vi "Main.vi"() -> ()   [LabVIEW 2014]
doc: "该连续测量范例项目在队列消息处理器模板的基础上实现。\n\n事件处理循环负责按用户界面操作生成对应的消息。\n\n消息处理循环负责对事件处理循环或其他消息生成的消息进行处理。其中还包括用于采集和记录消息处理循环的子VI，以及用于更新图表的循环。"
uses:
  Settings/Settings.ctl
  Acquisition/Hardware Configuration.ctl
  Acquisition/Signal Type.ctl
  Logging/Logging Configuration.ctl
  controls/UI Data.ctl
  controls/UI State.ctl
  support/Message Queue/Enqueue Message (Single).vi
  support/Message Queue/Enqueue Message (Array).vi
  <vilib>/Utility/error.llb/Error Cluster From Error Code.vi
  <vilib>/ErrorRing/Error Ring.xnode
  Acquisition/Acquisition.lvlib
  Logging/Logging.lvlib
  Settings/Settings.lvlib
  support/User Event - Stop/User Event - Stop.lvlib
  support/Message Queue/Message Queue.lvlib
panel:
  out "数据":waveform(dbl)[](graph)
  in  "设置":bool
  in  "开始":bool
  in  "停止":bool
  out "状态":string
  in  "退出":bool
  # "连续测量数据记录器"
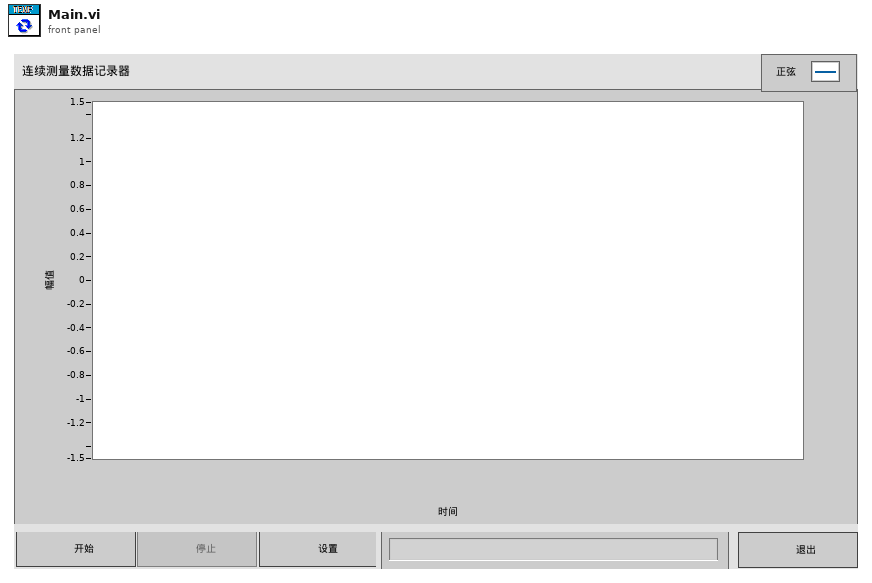
[diagram p1: front panel]
types:
  T1 = typedef "UI State.ctl" = enum16{"Idle", "Acquiring and Logging", "Waiting for Exit", "Waiting for Exit (Acq Stopped)", "Waiting for Exit (Log Stopped)", "Waiting for Stop", "Waiting for Stop (Acq Stopped)", "Waiting for Stop (Log Stopped)"}
  T2 = typedef "UI Data.ctl" = cluster{"开始引用":refnum<vi>, "停止引用":refnum<vi>, "设置引用":refnum<vi>, "退出引用":refnum<vi>, "状态引用":refnum<vi>, "数据引用":refnum<vi>}
  T3 = typedef "Settings.lvlib/Settings.ctl" = cluster{"硬件配置":T4, "记录配置":T6}
  T4 = typedef "Acquisition.lvlib/Hardware Configuration.ctl" = cluster{"硬件引用句柄<替换此项>":string, "信号类型<替换该项>":T5}
  T5 = typedef "Acquisition.lvlib/Signal Type.ctl" = enum16{"Sine Wave", "Square with Noise"}
  T6 = typedef "Logging.lvlib/Logging Configuration.ctl" = cluster{"记录文件基路径":path, "TDMS文件引用":refnum<k34>}
  T7 = typedef "Message Queue.lvlib/All Message Queues.ctl" = cluster{"UI":refnum<queue>, "采集":refnum<queue>, "记录":refnum<queue>}
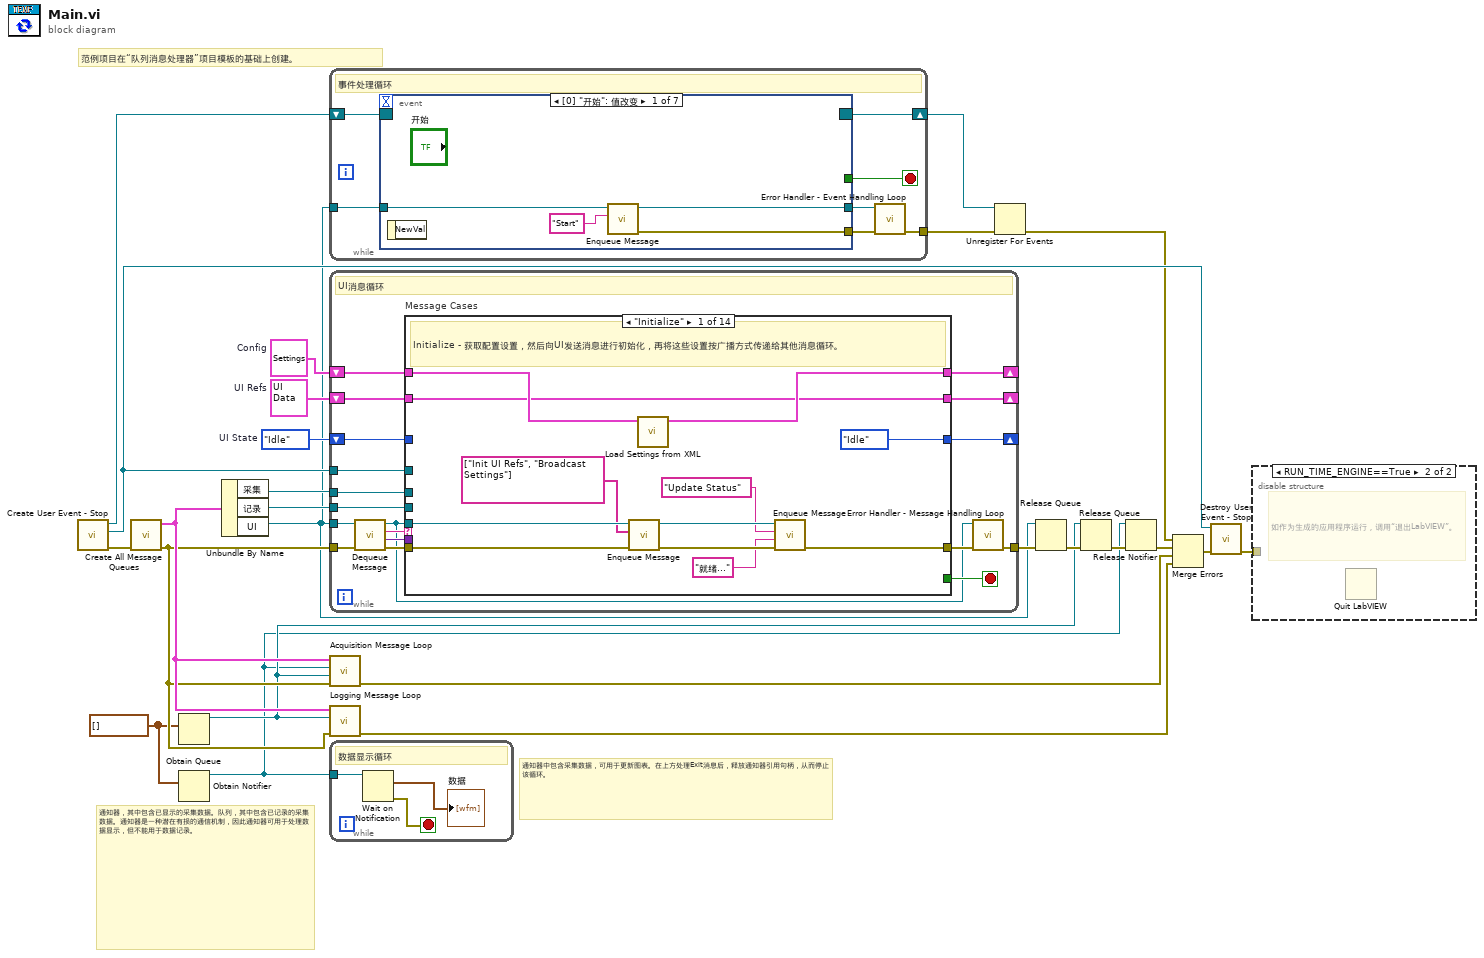
[diagram p0: block diagram]
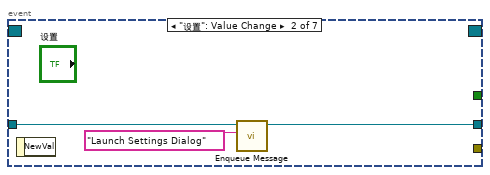
[diagram p3: hidden frame]
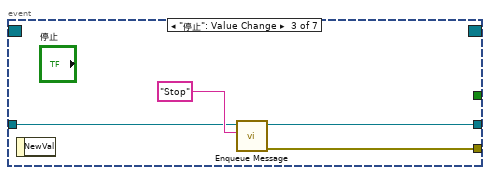
[diagram p4: hidden frame]
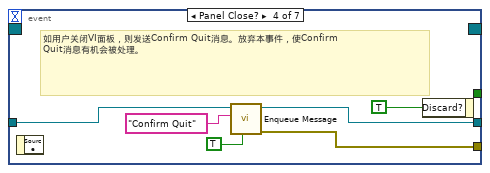
[diagram p5: hidden frame]
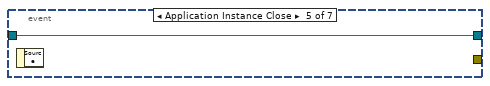
[diagram p6: hidden frame]
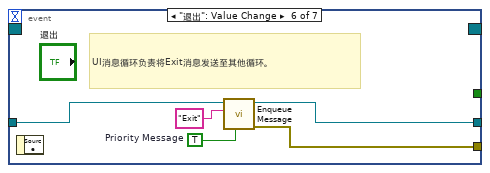
[diagram p7: hidden frame]
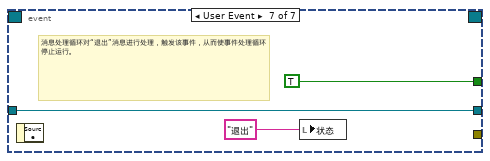
[diagram p8: hidden frame]
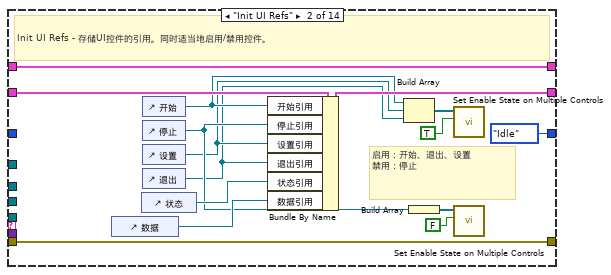
[diagram p9: hidden frame]
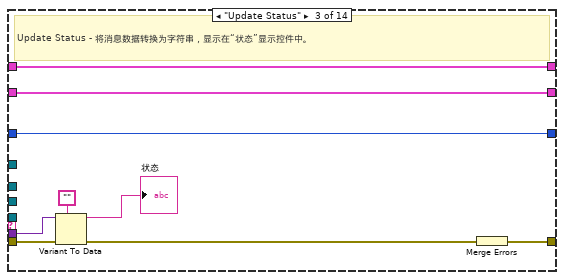
[diagram p10: hidden frame]
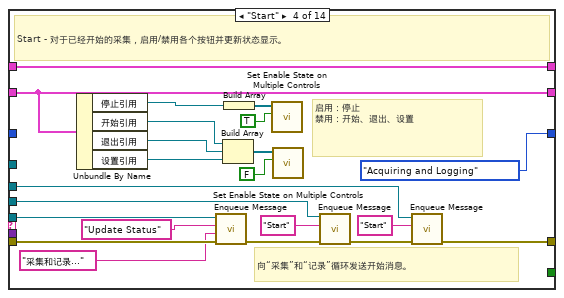
[diagram p11: hidden frame]
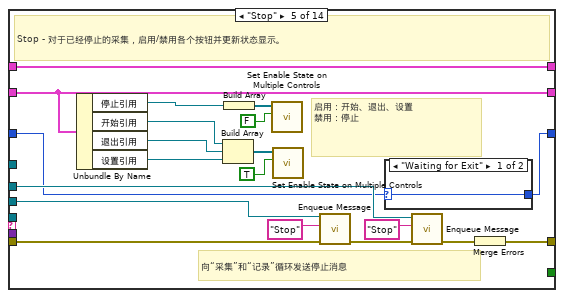
[diagram p12: hidden frame]
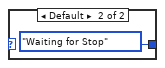
[diagram p13: hidden frame]
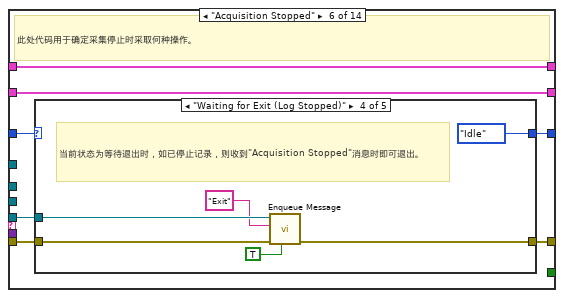
[diagram p14: hidden frame]
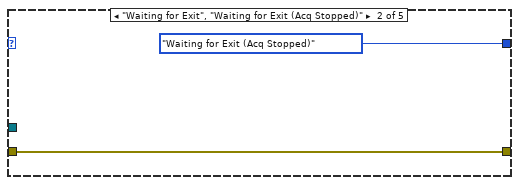
[diagram p16: hidden frame]
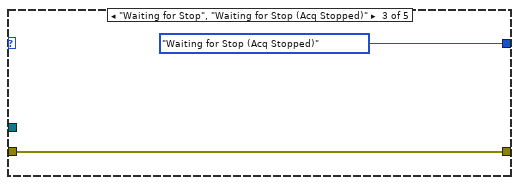
[diagram p17: hidden frame]
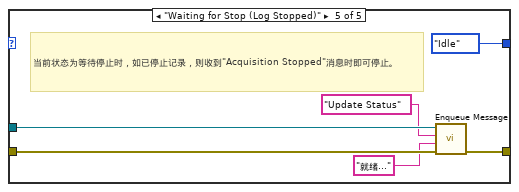
[diagram p18: hidden frame]
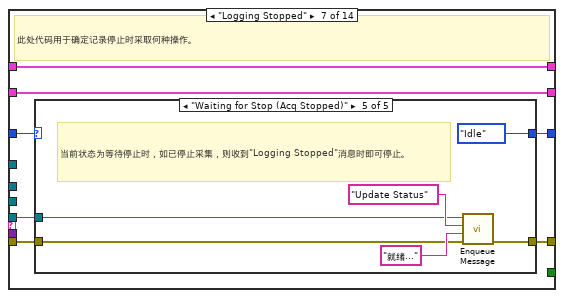
[diagram p19: hidden frame]
diagram:
  w10 = UI_State."Idle"  # UI State
  w1 = waveform(dbl)[] []
  w13 = T2 {"开始引用"=refnum, "停止引用"=refnum, "设置引用"=refnum, "退出引用"=refnum, "状态引用"=refnum, "数据引用"=refnum}  # UI Refs
  w16 = T3 {"硬件配置"={"硬件引用句柄<替换此项>"="", "信号类型<替换该项>"=enum."Sine Wave"}, "记录配置"={"记录文件基路径"=path "", "TDMS文件引用"=refnum}}  # Config
  # "范例项目在“队列消息处理器”项目模板的基础上创建。"
  # "通知器，其中包含已显示的采集数据。队列，其中包含已记录的采集数据。通知器是一种潜在有损的通信机制，因此通知器可用于处理数据显示，但不能用于数据记录。"
  # "通知器中包含采集数据，可用于更新图表。在上方处理Exit消息后，释放通知器引用句柄，从而停止该循环。"
  n1 = call "Create User Event - Stop.vi"() -> ("error out"=w20:cluster{"状态":bool, "代码":i32, "源":string}, "用户事件－停止"=w22:refnum<user-event>, "停止事件注册引用句柄"=w23:refnum<event-registration>)  [unwired: 9 in]
  n2 = call "Create All Message Queues.vi"("error in (no error)"=w20) -> ("error out"=w17:cluster{"状态":bool, "代码":i32, "源":string}, "消息队列输出"=w19:T7)  [unwired: 9 in]
  n3 = Obtain Queue(element data type=w1) -> (queue out=w3:refnum<queue>)  [unwired: 4 in, 2 out]
  n4 = Obtain Notifier(notification data type=w1) -> (notifier out=w2:refnum<notifier>)  [unwired: 3 in, 2 out]
  n5 = Unbundle By Name(w19) -> ("采集"=w12:refnum<queue>, "记录"=w11:refnum<queue>, "UI"=w8:refnum<queue>)
  n6 = while {
    tunnel: w8 -> [w31]
    tunnel: [w28] -> w24
    shift-right: [w30] -> w14
    shift-left: w23 -> [w32]
    stop <- w29 stop-if-true
    # "事件处理循环"
    n7 = event shown="[0] \"开始\": 值改变" {
      selector: w32 -> [_ _ _ _ _ _ _]
      dyn-events: [_ _ _ _ _ _ _] -> w30
      timeout: _ -> [_ _ _ _ _ _ _]
      tunnel: [_ _ _ _ _ _ TRUE ("Discard?")] -> w29
      tunnel: w31 -> [w36 w38 w42 w47 w50 w52 w56]
      tunnel: [w34 _ w41 w45 _ w55 _] -> w27
      tunnel: [w33 w37 w40 w46 w50 w51 w56] -> w26
      event "开始": Value Change {
        n8 = event-data() -> ()  [unwired: 1 in, 1 out]
        n9 = call-poly "Enqueue Message.vi"("消息"="Start" ("Message"), "消息队列"=w36) -> ("error out"=w34:cluster{"状态":bool, "代码":i32, "源":string}, "消息队列副本"=w33:refnum<queue>)  [unwired: 8 in]
      }
      event "设置": Value Change {
        n10 = event-data() -> ()  [unwired: 1 in, 1 out]
        n11 = call-poly "Enqueue Message.vi"("消息"="Launch Settings Dialog" ("Message"), "消息队列"=w38) -> ("消息队列副本"=w37:refnum<queue>)  [unwired: 8 in, 1 out]
      }
      event "停止": Value Change {
        n12 = event-data() -> ()  [unwired: 1 in, 1 out]
        n13 = call-poly "Enqueue Message.vi"("消息"="Stop" ("Message"), "消息队列"=w42) -> ("error out"=w41:cluster{"状态":bool, "代码":i32, "源":string}, "消息队列副本"=w40:refnum<queue>)  [unwired: 8 in]
      }
      event Panel Close? {
        # "如用户关闭VI面板，则发送Confirm Quit消息。放弃本事件，使Confirm Quit消息有机会被处理。"
        n14 = event-data() -> ()  [unwired: 1 in, 1 out]
        n15 = call-poly "Enqueue Message.vi"("优先消息？(F)"=TRUE ("Priority Message? (F)"), "消息"="Confirm Quit" ("Message"), "消息队列"=w47) -> ("error out"=w45:cluster{"状态":bool, "代码":i32, "源":string}, "消息队列副本"=w46:refnum<queue>)  [unwired: 7 in]
        n16 = event-data("Discard?"=TRUE) -> ()  [unwired: 1 in, 1 out]
      }
      event Application Instance Close {
        n17 = event-data() -> ()  [unwired: 1 in, 1 out]
      }
      event "退出": Value Change {
        w53 = TRUE  # Priority Message
        # "UI消息循环负责将Exit消息发送至其他循环。"
        n18 = event-data() -> ()  [unwired: 1 in, 1 out]
        n19 = call-poly "Enqueue Message.vi"("优先消息？(F)"=w53, "消息"="Exit" ("Message"), "消息队列"=w52) -> ("error out"=w55:cluster{"状态":bool, "代码":i32, "源":string}, "消息队列副本"=w51:refnum<queue>)  [unwired: 7 in]
      }
      event User Event {
        # "消息处理循环对“退出”消息进行处理，触发该事件，从而使事件处理循环停止运行。"
        n20 = event-data() -> ()  [unwired: 1 in, 1 out]
        n21 = local write "状态"("退出" ("Exit String")) -> ()
      }
    }
    n22 = call "Error Handler - Event Handling Loop.vi"("error in (no error)"=w27, "消息队列"=w26) -> ("错误输入副本"=w28:cluster{"状态":bool, "代码":i32, "源":string})  [unwired: 8 in, 1 out]
  }
  n23 = while {
    tunnel: w8 -> [w70]
    tunnel: w22 -> [w75]
    shift-right: [w69] -> _
    shift-left: w16 -> [w68]
    shift-right: [w66] -> _
    shift-left: w13 -> [w67]
    tunnel: w12 -> [w65]
    tunnel: w11 -> [w64]
    shift-right: [w59] -> _
    shift-left: w10 -> [w60]
    tunnel: w17 -> [w74]
    tunnel: [w63] -> w25
    stop <- w76 stop-if-true
    # "UI消息循环"
    n24 = call "Dequeue Message.vi"("error in (no error)"=w74, "消息队列"=w70) -> ("error out"=w73:cluster{"状态":bool, "代码":i32, "源":string}, "消息数据"=w71:variant, "消息"=w72:string, "消息队列副本"=w61:refnum<queue>)  [unwired: 6 in]
    n25 = case "Message Cases" shown="\"Initialize\"" w72 {
      selector: w72 -> [_ _ _ _ _ _ _ _ _ _ _ _ _ w292]
      tunnel: w61 -> [w80 _ _ w134 _ w159 w184 _ w224 w239 w248 _ _ _]
      tunnel: w73 -> [w79 w103 w111 w133 w153 w160 w185 w212 w226 _ w247 w273 w290 _]
      tunnel: [w84 w103 w112 w116 w154 w157 w182 w218 w219 w238 w246 w283 w289 w291] -> w62
      tunnel: [_ _ _ _ _ _ _ _ _ _ _ TRUE _ _] -> w76
      tunnel: w71 -> [_ _ w110 _ _ _ _ _ _ w240 _ _ _ _]
      tunnel: w75 -> [_ _ _ _ _ _ _ _ _ _ _ w284 _ _]
      tunnel: [w87 w102 w106 w132 w152 w163 w188 w216 w223 w244 w251 w282 w288 w295] -> w69
      tunnel: w68 -> [w88 w102 w106 w132 w152 w163 w188 w216 w227 w244 w251 w282 w288 w295]
      tunnel: w67 -> [w81 w101 w105 w129 w151 w162 w187 w210 w221 w243 w250 w281 w287 w294]
      tunnel: [w81 w98 w105 w129 w151 w162 w187 w210 w221 w243 w250 w281 w287 w294] -> w66
      tunnel: w65 -> [_ _ _ w115 w138 _ _ w209 _ _ _ w280 _ _]
      tunnel: w64 -> [_ _ _ w118 w141 _ _ w208 _ _ _ w279 _ _]
      tunnel: w60 -> [_ _ w104 _ w135 w161 w186 w207 w220 w236 w249 _ w286 w293]
      tunnel: [UI_State."Idle" ("UI State") UI_State."Idle" ("UI State") w104 UI_State."Acquiring and Logging" ("UI State") w136 w158 w183 w207 w220 w236 w245 UI_State."Idle" ("UI State") w286 w293] -> w59
      frame "Initialize" {
        # "Initialize - 获取配置设置，然后向UI发送消息进行初始化，再将这些设置按广播方式传递给其他消息循环。"
        n26 = call-poly "Enqueue Message.vi"("error in (no error)"=w79, "消息数组"=string[] ["Init UI Refs", "Broadcast Settings"], "消息队列"=w80) -> ("error out"=w86:cluster{"状态":bool, "代码":i32, "源":string}, "消息队列副本"=w85:refnum<queue>)  [unwired: 7 in]
        n27 = call "Load Settings from XML.vi"("设置输入"=w88) -> ("设置输出"=w87:T3)  [unwired: 9 in, 1 out]
        n28 = call-poly "Enqueue Message.vi"("error in (no error)"=w86, "消息数据"="就绪..." ("Ready..."), "消息"="Update Status" ("Message"), "消息队列"=w85) -> ("error out"=w84:cluster{"状态":bool, "代码":i32, "源":string})  [unwired: 6 in, 1 out]
      }
      frame "Init UI Refs" {
        # "启用：开始、退出、设置\n禁用：停止"
        # "Init UI Refs - 存储UI控件的引用。同时适当地启用/禁用控件。"
        n29 = control-ref of="数据"() -> (w99:refnum<vi>)
        n30 = control-ref of="状态"() -> (w100:refnum<vi>)
        n31 = control-ref of="开始"() -> (w92:refnum<vi>)
        n32 = control-ref of="停止"() -> (w93:refnum<vi>)
        n33 = control-ref of="设置"() -> (w91:refnum<vi>)
        n34 = control-ref of="退出"() -> (w90:refnum<vi>)
        n35 = Bundle By Name(cluster=w101, "开始引用"=w92, "停止引用"=w93, "设置引用"=w91, "退出引用"=w90, "状态引用"=w100, "数据引用"=w99) -> (w98:T2)
        n36 = Build Array(w92, w91, w90) -> (w96:refnum<vi>[])
        n37 = Build Array(w93) -> (w95:refnum<vi>[])
        n38 = call "Set Enable State on Multiple Controls.vi"("启用？"=TRUE ("Enable?"), "控件"=w96) -> ()  [unwired: 10 in]
        n39 = call "Set Enable State on Multiple Controls.vi"("启用？"=FALSE ("Enable?"), "控件"=w95) -> ()  [unwired: 10 in]
      }
      frame "Update Status" {
        # "Update Status - 将消息数据转换为字符串，显示在“状态”显示控件中。"
        n40 = Variant To Data(error in=w111, type="", Variant=w110) -> (data=→"状态":string, error out=w108:errorcluster)
        n41 = Merge Errors(w108) -> (w112:errorcluster)
      }
      frame "Start" {
        # "向“采集”和“记录”循环发送开始消息。"
        # "启用：停止\n禁用：开始、退出、设置"
        # "Start - 对于已经开始的采集，启用/禁用各个按钮并更新状态显示。"
        n42 = Unbundle By Name(w129) -> ("停止引用"=w124:refnum<vi>, "开始引用"=w123:refnum<vi>, "退出引用"=w122:refnum<vi>, "设置引用"=w121:refnum<vi>)
        n43 = call-poly "Enqueue Message.vi"("error in (no error)"=w133, "消息数据"="采集和记录..." ("Acquiring and Logging..."), "消息"="Update Status" ("Message"), "消息队列"=w134) -> ("error out"=w120:cluster{"状态":bool, "代码":i32, "源":string})  [unwired: 6 in, 1 out]
        n44 = Build Array(w123, w122, w121) -> (w127:refnum<vi>[])
        n45 = Build Array(w124) -> (w126:refnum<vi>[])
        n46 = call "Set Enable State on Multiple Controls.vi"("启用？"=TRUE ("Enable?"), "控件"=w126) -> ()  [unwired: 10 in]
        n47 = call "Set Enable State on Multiple Controls.vi"("启用？"=FALSE ("Enable?"), "控件"=w127) -> ()  [unwired: 10 in]
        n48 = call-poly "Enqueue Message.vi"("error in (no error)"=w120, "消息"="Start" ("Message"), "消息队列"=w118) -> ("error out"=w117:cluster{"状态":bool, "代码":i32, "源":string})  [unwired: 7 in, 1 out]
        n49 = call-poly "Enqueue Message.vi"("error in (no error)"=w117, "消息"="Start" ("Message"), "消息队列"=w115) -> ("error out"=w116:cluster{"状态":bool, "代码":i32, "源":string})  [unwired: 7 in, 1 out]
      }
      frame "Stop" {
        # "向“采集”和“记录”循环发送停止消息"
        # "启用：开始、退出、设置\n禁用：停止"
        # "Stop - 对于已经停止的采集，启用/禁用各个按钮并更新状态显示。"
        n50 = Unbundle By Name(w151) -> ("停止引用"=w146:refnum<vi>, "开始引用"=w145:refnum<vi>, "退出引用"=w144:refnum<vi>, "设置引用"=w143:refnum<vi>)
        n51 = Build Array(w145, w144, w143) -> (w149:refnum<vi>[])
        n52 = Build Array(w146) -> (w148:refnum<vi>[])
        n53 = call "Set Enable State on Multiple Controls.vi"("启用？"=FALSE ("Enable?"), "控件"=w148) -> ()  [unwired: 10 in]
        n54 = call "Set Enable State on Multiple Controls.vi"("启用？"=TRUE ("Enable?"), "控件"=w149) -> ()  [unwired: 10 in]
        n55 = call-poly "Enqueue Message.vi"("error in (no error)"=w153, "消息"="Stop" ("Message"), "消息队列"=w141) -> ("error out"=w140:cluster{"状态":bool, "代码":i32, "源":string})  [unwired: 7 in, 1 out]
        n56 = case shown="\"Waiting for Exit\"" w135 {
          selector: w135 -> [w155 _]
          tunnel: [w155 UI_State."Waiting for Stop" ("UI State")] -> w136
          frame "Waiting for Exit" {
          }
          frame Default {
          }
        }
        n57 = call-poly "Enqueue Message.vi"("error in (no error)"=w140, "消息"="Stop" ("Message"), "消息队列"=w138) -> ("error out"=w139:cluster{"状态":bool, "代码":i32, "源":string})  [unwired: 7 in, 1 out]
        n58 = Merge Errors(w139) -> (w154:errorcluster)
      }
      frame "Acquisition Stopped" {
        # "此处代码用于确定采集停止时采取何种操作。"
        n59 = case shown="\"Waiting for Exit (Log Stopped)\"" w161 {
          selector: w161 -> [w165 _ _ _ _]
          tunnel: w160 -> [w164 w167 w169 w175 w181]
          tunnel: w159 -> [_ _ _ w173 w178]
          tunnel: [w165 UI_State."Waiting for Exit (Acq Stopped)" ("UI State") UI_State."Waiting for Stop (Acq Stopped)" ("UI State") UI_State."Idle" ("UI State") UI_State."Idle" ("UI State")] -> w158
          tunnel: [w164 w167 w169 w174 w179] -> w157
          frame Default {
          }
          frame "Waiting for Exit", "Waiting for Exit (Acq Stopped)" {
          }
          frame "Waiting for Stop", "Waiting for Stop (Acq Stopped)" {
          }
          frame "Waiting for Exit (Log Stopped)" {
            # "当前状态为等待退出时，如已停止记录，则收到\"Acquisition Stopped\"消息时即可退出。"
            n60 = call-poly "Enqueue Message.vi"("优先消息？(F)"=TRUE ("Priority Message? (F)"), "error in (no error)"=w175, "消息"="Exit", "消息队列"=w173) -> ("error out"=w174:cluster{"状态":bool, "代码":i32, "源":string})  [unwired: 6 in, 1 out]
          }
          frame "Waiting for Stop (Log Stopped)" {
            # "当前状态为等待停止时，如已停止记录，则收到\"Acquisition Stopped\"消息时即可停止。"
            n61 = call-poly "Enqueue Message.vi"("error in (no error)"=w181, "消息数据"="就绪..." ("Ready..."), "消息"="Update Status" ("Message"), "消息队列"=w178) -> ("error out"=w179:cluster{"状态":bool, "代码":i32, "源":string})  [unwired: 6 in, 1 out]
          }
        }
      }
      frame "Logging Stopped" {
        # "此处代码用于确定记录停止时采取何种操作。"
        n62 = case shown="\"Waiting for Stop (Acq Stopped)\"" w186 {
          selector: w186 -> [w190 _ _ _ _]
          tunnel: w185 -> [w189 w192 w194 w200 w203]
          tunnel: w184 -> [_ _ _ w198 w202]
          tunnel: [w190 UI_State."Waiting for Exit (Log Stopped)" ("UI State") UI_State."Waiting for Stop (Log Stopped)" ("UI State") UI_State."Idle" ("UI State") UI_State."Idle" ("UI State")] -> w183
          tunnel: [w189 w192 w194 w199 w201] -> w182
          frame Default {
          }
          frame "Waiting for Exit", "Waiting for Exit (Log Stopped)" {
          }
          frame "Waiting for Stop", "Waiting for Stop (Log Stopped)" {
          }
          frame "Waiting for Exit (Acq Stopped)" {
            # "当前状态为等待退出时，如已停止采集，则收到\"Logging Stopped\"消息时即可退出。"
            n63 = call-poly "Enqueue Message.vi"("优先消息？(F)"=TRUE ("Priority Message? (F)"), "error in (no error)"=w200, "消息"="Exit", "消息队列"=w198) -> ("error out"=w199:cluster{"状态":bool, "代码":i32, "源":string})  [unwired: 6 in, 1 out]
          }
          frame "Waiting for Stop (Acq Stopped)" {
            # "当前状态为等待停止时，如已停止采集，则收到\"Logging Stopped\"消息时即可停止。"
            n64 = call-poly "Enqueue Message.vi"("error in (no error)"=w203, "消息数据"="就绪..." ("Ready..."), "消息"="Update Status" ("Message"), "消息队列"=w202) -> ("error out"=w201:cluster{"状态":bool, "代码":i32, "源":string})  [unwired: 6 in, 1 out]
          }
        }
      }
      frame "Broadcast settings" {
        w211 = "Update Settings" ("Message")
        # "Broadcast settings - 向“记录和采集”消息队列发送“更新设置”消息。"
        n65 = Unbundle By Name(w216) -> ("硬件配置"=w215:T4, "记录配置"=w214:T6)
        n66 = call-poly "Enqueue Message.vi"("消息数据"=w215, "消息"=w211, "消息队列"=w209) -> ("error out"=w217:cluster{"状态":bool, "代码":i32, "源":string})  [unwired: 7 in, 1 out]
        n67 = call-poly "Enqueue Message.vi"("error in (no error)"=w217, "消息数据"=w214, "消息"=w211, "消息队列"=w208) -> ("error out"=w213:cluster{"状态":bool, "代码":i32, "源":string})  [unwired: 6 in, 1 out]
        n68 = Merge Errors(w213, w212) -> (w218:errorcluster)
      }
      frame "Launch Settings Dialog" {
        # "Launch Settings Dialog - 用户单击“设置”按钮时，启动设置对话框。"
        n69 = call "Settings Dialog.vi"("error in (no error)"=w226, "设置输入"=w227) -> ("error out"=w222:cluster{"状态":bool, "代码":i32, "源":string}, "取消？"=w225:bool, "设置输出"=w223:T3)  [unwired: 6 in, 1 out]
        n70 = case shown="假" w225 {
          tunnel: w224 -> [w231 _]
          tunnel: w222 -> [w230 w232]
          tunnel: [w229 w232] -> w219
          frame False {
            n71 = call-poly "Enqueue Message.vi"("error in (no error)"=w230, "消息"="Broadcast Settings" ("Message"), "消息队列"=w231) -> ("error out"=w229:cluster{"状态":bool, "代码":i32, "源":string})  [unwired: 7 in, 1 out]
          }
          frame True {
          }
        }
      }
      frame "Error" {
        # "始终转换错误数据，包括即将发生的错误。"
        # "Error - 检查错误消息数据及其响应。本应用程序中，该消息由每个循环结束处的“错误处理”VI发送。"
        n72 = Variant To Data(type=errorcluster {"status"=FALSE, "code"=0, "source"=""} ("error constant"), Variant=w240) -> (data=w235:errorcluster, error out=w241:errorcluster)  [unwired: 1 in]
        n73 = call <vilib>:"Simple Error Handler.vi"("error in (no error)"=w235) -> ()  [unwired: 4 in, 5 out]
        n74 = call-poly "Enqueue Message.vi"("优先消息？(F)"=TRUE ("Priority Message? (F)"), "消息"="Exit", "消息队列"=w239) -> ("error out"=w237:cluster{"状态":bool, "代码":i32, "源":string})  [unwired: 7 in, 1 out]
        n75 = Merge Errors(w237, w241) -> (w238:errorcluster)
      }
      frame "Confirm Quit" {
        # "Confirm Quit - 该消息用于确认用户是否需要退出应用程序。"
        n76 = case shown="\"Acquiring and Logging\"" w249 {
          tunnel: w248 -> [w257 w261]
          tunnel: w247 -> [w256 w260]
          tunnel: [w255 w259] -> w246
          tunnel: [UI_State."Idle" ("UI State") w258] -> w245
          frame Default {
            # "如收到'Confirm Quit'消息时系统处于空闲状态，则不需要弹出确认提示。"
            n77 = call-poly "Enqueue Message.vi"("优先消息？(F)"=TRUE ("Priority Message? (F)"), "error in (no error)"=w256, "消息"="Exit", "消息队列"=w257) -> ("error out"=w255:cluster{"状态":bool, "代码":i32, "源":string})  [unwired: 6 in, 1 out]
          }
          frame "Acquiring and Logging" {
            n78 = Two Button Dialog(message="采集仍在执行中，是否确定退出？" ("Confirm Quit Message"), 1:"否" ("No"), 2:"是" ("Yes")) -> (T button?=w262:bool)
            n79 = case shown="真" w262 {
              tunnel: w261 -> [_ w271]
              tunnel: w260 -> [w267 w272]
              tunnel: [w267 w270] -> w259
              tunnel: [UI_State."Acquiring and Logging" ("UI State") UI_State."Waiting for Exit" ("UI State")] -> w258
              frame False {
                # "用户不希望退出。"
              }
              frame True {
                n80 = call-poly "Enqueue Message.vi"("error in (no error)"=w272, "消息"="Stop", "消息队列"=w271) -> ("error out"=w270:cluster{"状态":bool, "代码":i32, "源":string})  [unwired: 7 in, 1 out]
              }
            }
          }
        }
      }
      frame "Exit" {
        w275 = TRUE ("Priority Message? (F)")
        w276 = "Exit" ("Message")
        # "停止VI"
        # "Exit - 发送“退出”消息至采集和记录循环，并触发用户事件停止事件处理循环。"
        n81 = call-poly "Enqueue Message.vi"("优先消息？(F)"=w275, "error in (no error)"=w273, "消息"=w276, "消息队列"=w280) -> ("error out"=w277:cluster{"状态":bool, "代码":i32, "源":string})  [unwired: 6 in, 1 out]
        n82 = call-poly "Enqueue Message.vi"("优先消息？(F)"=w275, "error in (no error)"=w277, "消息"=w276, "消息队列"=w279) -> ("error out"=w274:cluster{"状态":bool, "代码":i32, "源":string})  [unwired: 6 in, 1 out]
        n83 = call "Fire User Event - Stop.vi"("error in (no error)"=w274, "用户事件－停止"=w284) -> ("error out"=w283:cluster{"状态":bool, "代码":i32, "源":string})  [unwired: 9 in]
      }
      frame "---Copy This Frame---" {
        # "如需创建新消息，可创建该帧的副本。在副本中，将本注释更改为对应消息的注释。"
        n84 = Merge Errors(w290) -> (w289:errorcluster)
      }
      frame Default {
        # "如得到的消息未经任何分支定义，则运行“默认”分支。输出程序错误。"
        n85 = xnode "Error Ring"("参数 0"=w292) -> ("错误输出"=w291:errorcluster)
      }
    }
    n86 = call "Error Handler - Message Handling Loop.vi"("error in (no error)"=w62, "消息队列"=w61) -> ("错误输入副本"=w63:cluster{"状态":bool, "代码":i32, "源":string})  [unwired: 8 in, 1 out]
  }
  n87 = call "Acquisition Message Loop.vi"("error in (no error)"=w17, "数据队列"=w3, "数据通知器"=w2, "消息队列"=w19) -> ("error out"=w21:cluster{"状态":bool, "代码":i32, "源":string})  [unwired: 7 in]
  n88 = call "Logging Message Loop.vi"("error in (no error)"=w17, "数据队列"=w3, "消息队列"=w19) -> ("error out"=w18:cluster{"状态":bool, "代码":i32, "源":string})  [unwired: 8 in]
  n89 = while "Data Display Loop" {
    tunnel: w2 -> [w305]
    stop <- w303 stop-if-true
    # "数据显示循环"
    n90 = Wait on Notification(notifier=w305) -> (notification=→"数据":waveform(dbl)[], error out=w303:errorcluster)  [unwired: 3 in, 2 out]
  }
  n91 = Unregister For Events(event registration refnum=w14, error in=w24) -> (error out=w15:errorcluster)
  n92 = Release Queue(queue=w8, error in (no error)=w25) -> (error out=w6:errorcluster)  [unwired: 1 in, 2 out]
  n93 = Release Queue(queue=w3, error in (no error)=w6) -> (error out=w5:errorcluster)  [unwired: 1 in, 2 out]
  n94 = Release Notifier(notifier=w2, error in (no error)=w5) -> (error out=w4:errorcluster)  [unwired: 1 in, 2 out]
  n95 = Merge Errors(w15, w4, w21, w18) -> (w9:errorcluster)
  n96 = call "Destroy User Event - Stop.vi"("error in (no error)"=w9, "用户事件－停止"=w22) -> ("error out"=w7:cluster{"状态":bool, "代码":i32, "源":string})  [unwired: 9 in]
  n97 = disable-structure shown="RUN_TIME_ENGINE==True" {
    disable-tunnel: w7 -> [_ _]
    frame condition #0 (active) {
    }
    frame condition #1 {
      # "如作为生成的应用程序运行，调用“退出LabVIEW”。"
      n98 = Quit LabVIEW() -> ()  [unwired: 1 in]
    }
  }
